vi "XIPIN_AXI_Memory_Mapped_To_PCI_Express_2_7.vi"   [LabVIEW 2017]
doc: "The Advanced eXtensible Interface (AXI) Root Port/Endpoint (RP/EP) Bridge for PCI Express is an interface between the AXI4 and PCI Express\n------------------------------------\n<b>Need License</b> : No\n<b>Interface</b> : AXI4"
uses:
  <vilib>/rvi/XilinxIP/XIPIN_XNode/niFpgaXIPIN.xnode
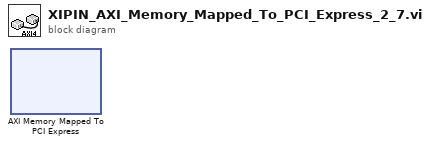
[diagram p0: block diagram]
diagram:
  n1 = xnode ("AXI Memory Mapped To PCI Express")() -> ()
